vi "PH_ImageOperator.PC CamType.vi"(0 "i ref in":refnum<vi>, 2 "Nearfield/Farfield":bool, 5 "error in (no error)":errorcluster) -> (14 "i ref out":refnum<vi>, 19 "error out":errorcluster)   [LabVIEW 2014, in "PH_ImageOperator.lvlib"]
doc: "This is the Action of the \"PositionOn\"-Case: It sets some attributes and GUI elements."
uses:
  PH_ImageOperator.lvlib
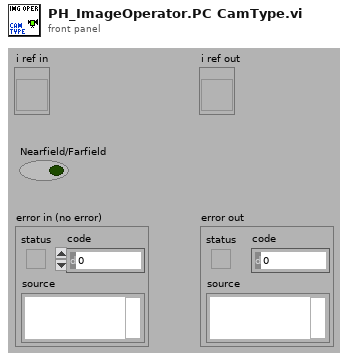
[diagram p1: front panel]
types:
  T1 = typedef "PH_ImageOperator.lvlib/PH_ImageOperator.i attribute.ctl" = cluster{"GUI Refs":cluster{"Delete":refnum<vi>, "Calibration status":refnum<vi>, "BI subtracted":refnum<vi>, "calc Energy":refnum<vi>, "Energy: expected value":refnum<vi>, "Energy: Tolerance":refnum<vi>, "Energy calculated":refnum<vi>, "Energy":refnum<vi>, "calc Beam Anal":refnum<vi>, "Maj Diam 1/esquare":refnum<vi>, "Min Diam 1/esquare":refnum<vi>, "Azi Angle":refnum<vi>, "Min/Maj Diam esquare":refnum<vi>, "Beam analysed":refnum<vi>, "CoG - x":refnum<vi>, "CoG - y":refnum<vi>, "BA: Method":refnum<vi>, "BA: Steps":refnum<vi>, "BA: Factor":refnum<vi>, "calc Traces":refnum<vi>, "Traces: Fit Gauss":refnum<vi>, "Traces calculated":refnum<vi>, "Maj FWHM":refnum<vi>, "Min FWHM":refnum<vi>, "Major Trace":refnum<vi>, "Minor Trace":refnum<vi>, "Maj Fit Order":refnum<vi>, "Min Fit Order":refnum<vi>, "Position calculated":refnum<vi>, "Position":refnum<vi>, "Type":refnum<vi>, "Center":refnum<vi>, "exp - X":refnum<vi>, "exp - Y":refnum<vi>, "Tolerance":refnum<vi>, "f":refnum<vi>, "M":refnum<vi>, "D":refnum<vi>, "q":refnum<vi>, "Dummy Method":refnum<vi>, "Dummy Type":refnum<vi>, "Global On":refnum<vi>, "Traces: No offset":refnum<vi>, "Maj 99%":refnum<vi>, "Min 99%":refnum<vi>, "GUI FF Image":refnum<vi>, "calc Fill Factor":refnum<vi>, "FF calculated":refnum<vi>, "Fill Factor: Filter?":refnum<vi>, "FF: Damage Threshold":refnum<vi>, "FF: Threshold":refnum<vi>, "FF: max allow. Energy":refnum<vi>, "FF: Fillfactor":refnum<vi>, "Calibration data":refnum<vi>}, "List of GUIs":string[], "Calibration":cluster{"Status":T2, "Calibration data":T3, "Calibration Data File":path}, "Final Image":cluster{"BI Subtraction Failure":bool}, "Energy":cluster{"on":bool, "expected value [mJ]":dbl, "Tolerance [%]":dbl, "State":T2, "Energy [mJ]":dbl, "Unit":string, "calculated @":timestamp}, "Beam Analysis":cluster{"on":bool, "Data":T4, "Method":bool, "Steps":i32, "Factor":i32, "ROI":cluster{"Left":i32, "Top":i32, "Right":i32, "Bottom":i32}, "analysed @":timestamp}, "Trace Analysis":cluster{"on":bool, "Fit on":bool, "Maj FWHM":dbl, "Min FWHM":dbl, "Maj Fit Order":i32, "Min Fit Order":i32, "No Offset":bool, "Maj 99%":dbl, "Min 99%":dbl, "Traces":cluster{"XScaleName":string, "Y Scale Minimum":sgl, "Y Scale Maximum":sgl, "X Scale Minimum":sgl, "X Scale Maximum":sgl, "Traces":cluster{"Index":sgl[], "Trace":dbl[]}[]}[], "analysed @":timestamp}, "Position Analysis":cluster{"on":bool, "exp - X":i32, "exp - Y":i32, "focal length [mm]":dbl, "Magnification":dbl, "Delta":dbl, "Theta":dbl, "Tolerance":dbl, "Type":bool, "analysed @":timestamp}, "Fill Factor":cluster{"on":bool, "Filter on?":bool, "Threshold":dbl, "Damage Threshold [J/cm²]":dbl, "Fillfactor":dbl, "Max. allowed Energy [J]":dbl, "calculated @":timestamp}, "Statistician Service ID":i32, "Images":cluster{"Background":T5, "OP":T5, "GUI":T5, "BA: ROI":T5, "Trace: Turn":T5, "FF: Main":T5, "FF: Help":T5, "PSDB: BG":T5, "PSDB: OP":T5, "PSDB: FF":T5}}
  T2 = typedef "PH_StatusHandler.lvlib/PH_StatusHandler.Status.ctl" = i16
  T3 = typedef "PH_ImageCalibrator.lvlib/PH_ImageCalibrator.Calibration Data.ctl" = cluster{"Date":string, "Time":string, "Cam Settings":cluster{"Cam ID":string, "Gain":dbl, "Brightness":dbl, "Shutter":dbl, "Cam Error":bool, "Mode":i32}, "Background Image":cluster{"Image":dbl[][], "Image Error":bool}, "Linear Calibration":cluster{"Calibration Factor":dbl, "not mm or mrad":bool}, "Energy Calibration":cluster{"Calibration Factor":dbl, "no mJ":bool}}
  T4 = typedef "PH_ImageOperator.lvlib/PH_ImageOperator.Beam Analysis Data.ctl" = cluster{"CoG-x":sgl, "CoG-y":sgl, "Maj Dim":dbl, "Min Dim":dbl, "Ellipticity":dbl, "Azimuth Angle [rad]":dbl, "Azi Angle rel to Maj?":bool}
  T5 = typedef "IMAQ Image.ctl" = refnum<image>
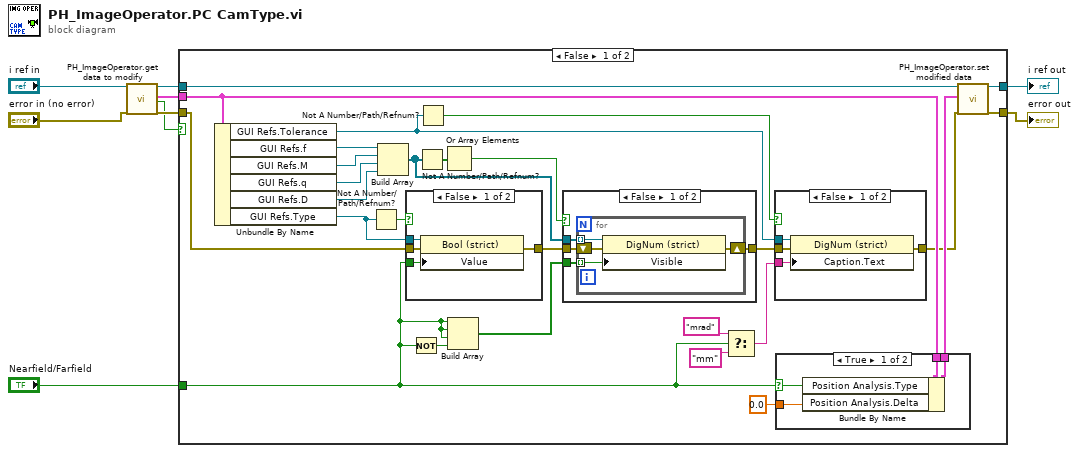
[diagram p0: block diagram]
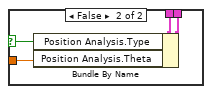
[diagram p2: hidden frame]
diagram:
  n1 = call "PH_ImageOperator.get data to modify.vi"("i ref in"="i ref in", "error in (no error)"="error in (no error)") -> ("i ref out"=w6:refnum<vi>, "i attribute"=w8:T1, "timed out"=w1:bool, "error out"=w4:errorcluster)  [unwired: 14 in]
  n2 = case shown="False" w1 {
    tunnel: "Nearfield/Farfield" -> [w11 _]
    tunnel: w8 -> [w32 _]
    tunnel: [w35 w65] -> w7
    tunnel: w6 -> [w34 w65]
    tunnel: [w33 w64] -> w5
    tunnel: w4 -> [w31 w64]
    frame False {
      n3 = Unbundle By Name(w32) -> ("GUI Refs.Tolerance"=w18:refnum<vi>, "GUI Refs.f"=w26:refnum<vi>, "GUI Refs.M"=w25:refnum<vi>, "GUI Refs.q"=w24:refnum<vi>, "GUI Refs.D"=w23:refnum<vi>, "GUI Refs.Type"=w29:refnum<vi>)
      n4 = Not A Number/Path/Refnum?(number/path/refnum=w29) -> (NaN/Path/Refnum?=w30:bool)
      n5 = Build Array(w26, w25, w24, w23) -> (w22:refnum<vi>[])
      n6 = case shown="False" w30 {
        tunnel: w29 -> [w62 _]
        tunnel: w11 -> [w61 _]
        tunnel: w31 -> [w60 w63]
        tunnel: [w59 w63] -> w28
        frame False {
          n7 = property class="Bool (strict)"(reference=w62, error in=w60, "Value"=w61) -> (error out=w59:errorcluster)  [unwired: 1 out]
        }
        frame True {
        }
      }
      n8 = Not(x=w11) -> (.not. x?=w20:bool)
      n9 = Not A Number/Path/Refnum?(number/path/refnum=w22) -> (NaN/Path/Refnum?=w27:bool[])
      n10 = Not A Number/Path/Refnum?(number/path/refnum=w18) -> (NaN/Path/Refnum?=w17:bool)
      n11 = Or Array Elements(Boolean array=w27) -> (logical OR=w21:bool)
      n12 = Build Array(w11, w11, w11, w20) -> (w14:bool[])
      n13 = case shown="False" w21 {
        tunnel: w22 -> [w53 _]
        tunnel: w14 -> [w52 _]
        tunnel: w28 -> [w51 w58]
        tunnel: [w50 w58] -> w19
        frame False {
          n14 = for {
            tunnel: w53 -> [w57] mode=indexing
            tunnel: w52 -> [w56] mode=indexing
            shift-right: [w54] -> w50
            shift-left: w51 -> [w55]
            n15 = property class="DigNum (strict)"(reference=w57, error in=w55, "Visible"=w56) -> (error out=w54:errorcluster)  [unwired: 1 out]
          }
        }
        frame True {
        }
      }
      n16 = Select(t="mrad", s=w11, f="mm") -> (s? t:f=w16:string)
      n17 = case shown="False" w17 {
        tunnel: w18 -> [w48 _]
        tunnel: w16 -> [w47 _]
        tunnel: w19 -> [w46 w49]
        tunnel: [w45 w49] -> w15
        frame False {
          n18 = property class="DigNum (strict)"(reference=w48, error in=w46, "Caption.Text"=w47) -> (error out=w45:errorcluster)  [unwired: 1 out]
        }
        frame True {
        }
      }
      n19 = case shown="True" w11 {
        selector: w11 -> [w38 w42]
        tunnel: [w40 w44] -> w36
        tunnel: w32 -> [w39 w43]
        tunnel: 0.0 ("Position Analysis.Theta") -> [w37 w41]
        frame True {
          n20 = Bundle By Name(cluster=w39, "Position Analysis.Type"=w38, "Position Analysis.Delta"=w37) -> (w40:T1)
        }
        frame False {
          n21 = Bundle By Name(cluster=w43, "Position Analysis.Type"=w42, "Position Analysis.Theta"=w41) -> (w44:T1)
        }
      }
      n22 = call "PH_ImageOperator.set modified data.vi"("i ref in"=w34, "i attribute"=w36, "error in (no error)"=w15) -> ("i ref out"=w35:refnum<vi>, "error out"=w33:errorcluster)  [unwired: 15 in]
    }
    frame True {
    }
  }
  "i ref out" <- w7
  "error out" <- w5
